vi "Menu Callback.vi"(11 "Receiver":refnum<class "LQObject.lvclass">) -> ()   [LabVIEW 2014, in "Dual Mode Thermometer.lvclass"]
doc: "Callback VI: Called when the user clicks the \"Display Temperature...\" menu item.\n\n\nCopyright (c) 2019 Sze Howe Koh.\nThis code is licensed under the MIT license."
uses:
  Dual Mode Thermometer.lvclass
  <vilib>/addons/LQ/LQ Core/LQObject/LQObject.lvclass
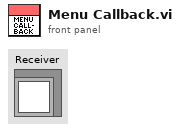
[diagram p1: front panel]
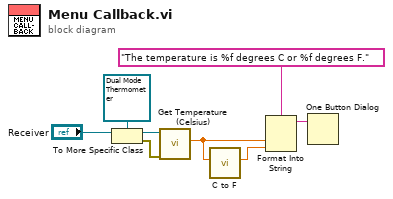
[diagram p0: block diagram]
diagram:
  n1 = To More Specific Class(target class=refnum<class "Dual Mode Thermometer.lvclass"> refnum ("Dual Mode Thermometer"), reference="Receiver") -> (specific class reference=w4:refnum<class "Dual Mode Thermometer.lvclass">, error out=w3:errorcluster)  [unwired: 1 in]
  n2 = call "Get Temperature (Celsius).vi"("Error In"=w3, "Dual Mode Thermometer in"=w4) -> ("Temperature (Celsius)"=w2:dbl)  [unwired: 7 in, 2 out]
  n3 = call "C to F.vi"("Value [°C]"=w2) -> ("Value [°F]"=w1:dbl)  [unwired: 10 in]
  n4 = Format Into String(format string="The temperature is %f degrees C or %f degrees F.", w2, w1) -> (resulting string=w8:string)  [unwired: 2 in, 1 out]
  n5 = One Button Dialog(message=w8) -> ()  [unwired: 1 in, 1 out]
